vi "EGG Analysis.vi"() -> ()   [LabVIEW 2020]
uses:
  <vilib>/sound2/lvsound2.llb/Sound File Read Open.vi
  <vilib>/sound2/lvsound2.llb/Sound File Read (DBL).vi
  <vilib>/Waveform/WDTOps.llb/WDT Get Waveform Subset DBL.vi
  <vilib>/measure/matone.llb/Extract Multiple Tone Information 1 Chan.vi
  <vilib>/measure/NI_MAPro.lvlib
  <vilib>/Analysis/NI_AALPro.lvlib
panel:
  in  "OK Button":bool
  out "Sample Subset":waveform(dbl)(graph)
  out "Full Sample":waveform(dbl)(graph)
  in  "Cutoff":dbl=0.01 min=0.01 max=0.99 step=0.01
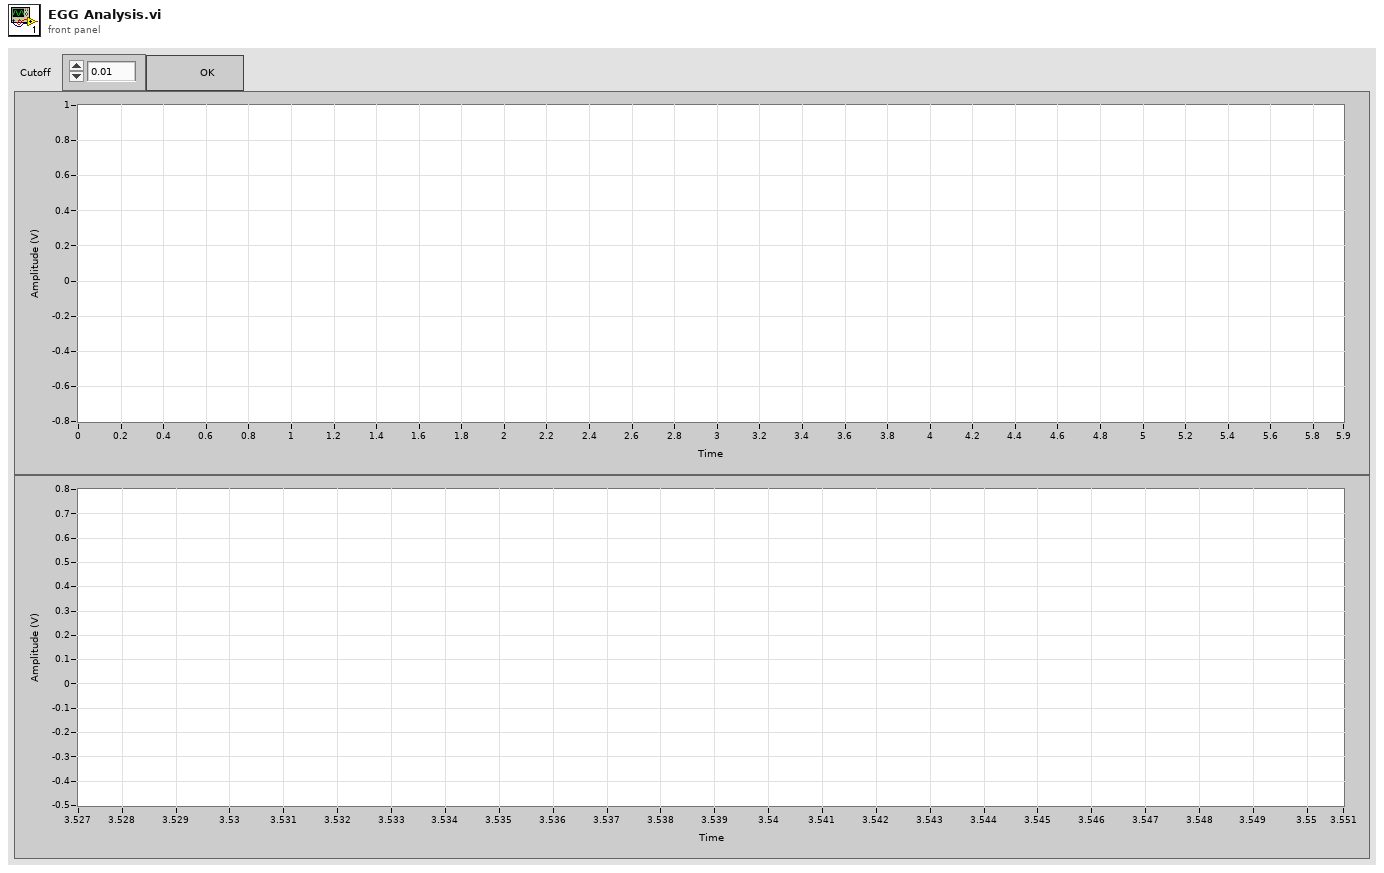
[diagram p1: front panel]
types:
  T1 = typedef "Sound File Refnum.ctl" = refnum<file>
  T2 = cluster{"Name":string, "Color":u32, "Style":u8, "Point Style":u8, "Name Visible":bool, "Allow Drag":bool, "Cursor Mode":u32, "Plot":i32, "Index":i32, "Position":cluster{"X":dbl, "Y":dbl}, "X Scale":u32, "Y Scale":u32, "Watch Plots":i32[], "Watch All Plots":bool, "Plot Area":i32, "Label Offset":cluster{"X":dbl, "Y":dbl}}[]
  T3 = typedef "LVCursorListTypeDef.ctl" = cluster{"Name":string, "Color":u32, "Style":u8, "Point Style":u8, "Name Visible":bool, "Allow Drag":bool, "Cursor Mode":u32, "Plot":i32, "Index":i32, "Position":cluster{"X":dbl, "Y":dbl}, "X Scale":u32, "Y Scale":u32, "Watch Plots":i32[], "Watch All Plots":bool, "Plot Area":i32, "Label Offset":cluster{"X":dbl, "Y":dbl}}[]
  T4 = cluster{"CrsrList[0]":cluster{"Name":string, "Color":u32, "Style":u8, "Point Style":u8, "Name Visible":bool, "Allow Drag":bool, "Cursor Mode":u32, "Plot":i32, "Index":i32, "Position":cluster{"X":dbl, "Y":dbl}, "X Scale":u32, "Y Scale":u32, "Watch Plots":i32[], "Watch All Plots":bool, "Plot Area":i32, "Label Offset":cluster{"X":dbl, "Y":dbl}}, "CrsrList[1]":cluster{"Name":string, "Color":u32, "Style":u8, "Point Style":u8, "Name Visible":bool, "Allow Drag":bool, "Cursor Mode":u32, "Plot":i32, "Index":i32, "Position":cluster{"X":dbl, "Y":dbl}, "X Scale":u32, "Y Scale":u32, "Watch Plots":i32[], "Watch All Plots":bool, "Plot Area":i32, "Label Offset":cluster{"X":dbl, "Y":dbl}}, "CrsrList[2]":cluster{"Name":string, "Color":u32, "Style":u8, "Point Style":u8, "Name Visible":bool, "Allow Drag":bool, "Cursor Mode":u32, "Plot":i32, "Index":i32, "Position":cluster{"X":dbl, "Y":dbl}, "X Scale":u32, "Y Scale":u32, "Watch Plots":i32[], "Watch All Plots":bool, "Plot Area":i32, "Label Offset":cluster{"X":dbl, "Y":dbl}}, "CrsrList[3]":cluster{"Name":string, "Color":u32, "Style":u8, "Point Style":u8, "Name Visible":bool, "Allow Drag":bool, "Cursor Mode":u32, "Plot":i32, "Index":i32, "Position":cluster{"X":dbl, "Y":dbl}, "X Scale":u32, "Y Scale":u32, "Watch Plots":i32[], "Watch All Plots":bool, "Plot Area":i32, "Label Offset":cluster{"X":dbl, "Y":dbl}}, "CrsrList[4]":cluster{"Name":string, "Color":u32, "Style":u8, "Point Style":u8, "Name Visible":bool, "Allow Drag":bool, "Cursor Mode":u32, "Plot":i32, "Index":i32, "Position":cluster{"X":dbl, "Y":dbl}, "X Scale":u32, "Y Scale":u32, "Watch Plots":i32[], "Watch All Plots":bool, "Plot Area":i32, "Label Offset":cluster{"X":dbl, "Y":dbl}}, "CrsrList[5]":cluster{"Name":string, "Color":u32, "Style":u8, "Point Style":u8, "Name Visible":bool, "Allow Drag":bool, "Cursor Mode":u32, "Plot":i32, "Index":i32, "Position":cluster{"X":dbl, "Y":dbl}, "X Scale":u32, "Y Scale":u32, "Watch Plots":i32[], "Watch All Plots":bool, "Plot Area":i32, "Label Offset":cluster{"X":dbl, "Y":dbl}}, "CrsrList[6]":cluster{"Name":string, "Color":u32, "Style":u8, "Point Style":u8, "Name Visible":bool, "Allow Drag":bool, "Cursor Mode":u32, "Plot":i32, "Index":i32, "Position":cluster{"X":dbl, "Y":dbl}, "X Scale":u32, "Y Scale":u32, "Watch Plots":i32[], "Watch All Plots":bool, "Plot Area":i32, "Label Offset":cluster{"X":dbl, "Y":dbl}}, "CrsrList[7]":cluster{"Name":string, "Color":u32, "Style":u8, "Point Style":u8, "Name Visible":bool, "Allow Drag":bool, "Cursor Mode":u32, "Plot":i32, "Index":i32, "Position":cluster{"X":dbl, "Y":dbl}, "X Scale":u32, "Y Scale":u32, "Watch Plots":i32[], "Watch All Plots":bool, "Plot Area":i32, "Label Offset":cluster{"X":dbl, "Y":dbl}}, "CrsrList[8]":cluster{"Name":string, "Color":u32, "Style":u8, "Point Style":u8, "Name Visible":bool, "Allow Drag":bool, "Cursor Mode":u32, "Plot":i32, "Index":i32, "Position":cluster{"X":dbl, "Y":dbl}, "X Scale":u32, "Y Scale":u32, "Watch Plots":i32[], "Watch All Plots":bool, "Plot Area":i32, "Label Offset":cluster{"X":dbl, "Y":dbl}}}
  T5 = cluster{"detected frequency":dbl, "detected amplitude":dbl, "detected phase (deg)":dbl}[]
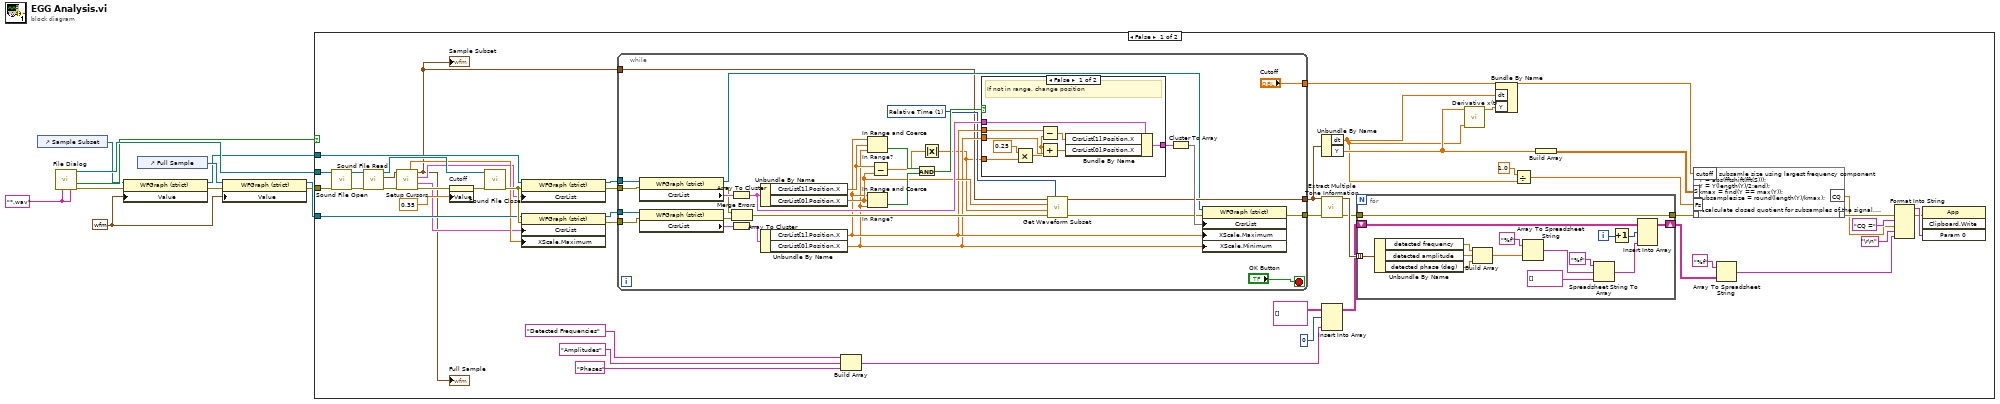
[diagram p0: block diagram]
diagram:
  w1 = waveform(dbl) {"t0"=timestamp(0 s since 1904-01-01), "dt"=1.0, "Y"=[]} ("Waveform")
  w10 = "*.wav" ("pattern (all files)")
  n1 = control-ref of="Sample Subset"() -> (w8:refnum<vi>)
  n2 = call "File Dialog"("pattern (all files)"=w10, "pattern label"=w10) -> ("selected path"=w11:path, "cancelled"=w9:bool, "error out"=w2:errorcluster)  [unwired: 10 in, 1 out]
  n3 = property class="WFGraph (strict)"(reference=w8, error in=w2, "Value"=w1) -> (reference out=w3:refnum<vi>, error out=w4:errorcluster)
  n4 = control-ref of="Full Sample"() -> (w7:refnum<vi>)
  n5 = property class="WFGraph (strict)"(reference=w7, error in=w4, "Value"=w1) -> (reference out=w6:refnum<vi>, error out=w5:errorcluster)
  n6 = case shown="False" w9 {
    tunnel: w11 -> [w58 _]
    tunnel: w5 -> [w57 _]
    tunnel: w3 -> [w42 _]
    tunnel: w6 -> [w41 _]
    frame False {
      n7 = call-poly <vilib>:"Sound File Open.vi"("error in (no error)"=w57, "path"=w58) -> ("error out"=w60:errorcluster, "sound file refnum"=w59:T1)  [unwired: 8 in]
      n8 = call-poly <vilib>:"Sound File Read.vi"("error in (no error)"=w60, "sound file refnum"=w59) -> ("error out"=w46:errorcluster, "data"=w54:waveform(dbl)[], "sound file refnum out"=w53:T1)  [unwired: 5 in, 2 out]
      n9 = call "Setup Cursors.vi"("error in (no error)"=w46, "data"=w54) -> ("error out"=w44:errorcluster, "Cursor List 2"=w33:T2, "Cursor List"=w34:T2, "waveform out"=w32:waveform(dbl), "duration"=w35:dbl)  [unwired: 5 in]
      "Full Sample" <- w32
      "Sample Subset" <- w32
      n10 = property on="Cutoff" class="DigNum (strict)"(error in=w44, "Value"=0.35 ("Cutoff")) -> (error out=w43:errorcluster)  [unwired: 1 in, 1 out]
      n11 = call <vilib>:"Sound File Close.vi"("error in (no error)"=w43, "sound file refnum"=w53) -> ("error out"=w51:errorcluster)  [unwired: 9 in]
      n12 = property on="Property Node" class="WFGraph (strict)"(reference=w42, error in=w51, "CrsrList"=w34) -> (reference out=w49:refnum<vi>, error out=w50:errorcluster)
      n13 = property on="Property Node" class="WFGraph (strict)"(reference=w41, error in=w51, "CrsrList"=w33, "XScale.Maximum"=w35) -> (reference out=w48:refnum<vi>, error out=w47:errorcluster)
      n14 = while {
        tunnel: w32 -> [w77]
        tunnel: [w90] -> w40
        tunnel: ["Cutoff"] -> w52
        tunnel: [w83] -> w39
        tunnel: w50 -> [w82]
        tunnel: w49 -> [w81]
        tunnel: w48 -> [w80]
        tunnel: w47 -> [w79]
        stop <- "OK Button" stop-if-true
        w85 = u16 1 items=["Samples", "Relative Time"] ("start/duration format")
        n15 = property on="Property Node" class="WFGraph (strict)"(reference=w81, error in=w82) -> (reference out=w88:refnum<vi>, error out=w93:errorcluster, "CrsrList"=w105:T3)
        n16 = property on="Property Node" class="WFGraph (strict)"(reference=w80, error in=w79) -> (error out=w92:errorcluster, "CrsrList"=w104:T3)  [unwired: 1 out]
        n17 = Array To Cluster(array=w105) -> (cluster=w100:T4)
        n18 = Array To Cluster(array=w104) -> (cluster=w103:T4)
        n19 = Merge Errors(w93, w92) -> (w91:errorcluster)
        n20 = Unbundle By Name(w100) -> ("CrsrList[1].Position.X"=w95:dbl, "CrsrList[0].Position.X"=w94:dbl)
        n21 = Unbundle By Name(w103) -> ("CrsrList[1].Position.X"=w87:dbl, "CrsrList[0].Position.X"=w86:dbl)
        n22 = In Range and Coerce "In Range?"(upper limit=w87, x=w95, lower limit=w86) -> (In Range?=w99:bool)  [unwired: 1 out]
        n23 = In Range and Coerce "In Range?"(upper limit=w87, x=w94, lower limit=w86) -> (In Range?=w98:bool)  [unwired: 1 out]
        n24 = Subtract(x=w95, y=w94) -> (x-y=w96:dbl)
        n25 = And(x=w99, y=w98) -> (x .and. y?=w97:bool)
        n26 = Absolute Value(x=w96) -> (abs(x)=w76:dbl)
        n27 = case shown="False" w97 {
          tunnel: [w114 w115] -> w101
          tunnel: w100 -> [w113 w115]
          tunnel: w86 -> [w112 _]
          tunnel: w87 -> [w111 _]
          tunnel: w76 -> [w106 _]
          frame False {
            # "If not in range, change position"
            n28 = Multiply(x=0.25, y=w106) -> (x*y=w108:dbl)
            n29 = Subtract(x=w111, y=w108) -> (x-y=w110:dbl)
            n30 = Add(x=w108, y=w112) -> (x+y=w109:dbl)
            n31 = Bundle By Name(cluster=w113, "CrsrList[1].Position.X"=w110, "CrsrList[0].Position.X"=w109) -> (w114:T4)
          }
          frame True {
            # "Cursors are within bounds"
          }
        }
        n32 = call-poly <vilib>:"Get Waveform Subset.vi"("start/duration format"=w85, "error in (no error)"=w91, "duration"=w76, "start samples/time"=w94, "waveform in"=w77) -> ("error out"=w84:errorcluster, "waveform out"=w90:waveform(dbl))  [unwired: 1 in, 2 out]
        n33 = Cluster To Array(cluster=w101) -> (array=w102:T2)
        n34 = property on="Property Node" class="WFGraph (strict)"(reference=w88, error in=w84, "CrsrList"=w102, "XScale.Maximum"=w87, "XScale.Minimum"=w86) -> (error out=w83:errorcluster)  [unwired: 1 out]
      }
      n35 = Build Array("Detected Frequencies", "Amplitudes", "Phases") -> (w20:string[])
      n36 = Unbundle By Name(w40) -> ("dt"=w12:dbl, "Y"=w14:dbl[])
      n37 = call-poly <vilib>:"Extract Multiple Tone Information.vi"("time signal in"=w40, "error in (no error)"=w39) -> ("multiple tone information"=w37:T5, "error out"=w36:errorcluster)  [unwired: 11 in, 1 out]
      n38 = Insert Into Array(array=string[][] [], index (row)=0 ("disabled index (col)"), new element=w20) -> (w19:string[][])  [unwired: 1 in]
      n39 = for {
        tunnel: w37 -> [w75] mode=indexing
        tunnel: w36 -> [w74]
        tunnel: [w74] -> w30
        shift-right: [w72] -> w18
        shift-left: w19 -> [w73]
        i -> [w71]
        n40 = Unbundle By Name(w75) -> ("detected frequency"=w69:dbl, "detected amplitude"=w68:dbl, "detected phase (deg)"=w67:dbl)
        n41 = Build Array(w69, w68, w67) -> (w64:dbl[])
        n42 = Array To Spreadsheet String(array=w64, 3:"%f" ("format string")) -> (spreadsheet string=w65:string)  [unwired: 1 in]
        n43 = Spreadsheet String To Array(format string="%f", spreadsheet string=w65, array type (2D Dbl)=string[] []) -> (array=w62:string[])  [unwired: 1 in]
        n44 = Increment(x=w71) -> (x+1=w61:i32)
        n45 = Insert Into Array(array=w73, index (row)=w61, new element=w62) -> (w72:string[][])  [unwired: 1 in]
      }
      n46 = call <vilib>:"Derivative x(t).vi"("dt"=w12, "X"=w14) -> ("dX/dt"=w13:dbl[])  [unwired: 8 in, 1 out]
      n47 = Bundle By Name("dt"=w12, "Y"=w13) -> ()  [unwired: 1 in, 1 out]
      n48 = Divide(x=1.0, y=w12) -> (x/y=w38:dbl)
      n49 = Build Array(w14) -> (w55:dbl[][])
      n50 = script code="%find subsamle size using largest frequency component\nY = abs(fftshift(fft(S)));\nY = Y(length(Y)/2:end);\nkmax = find(Y == max(Y));\nsubsamplesize = round(length(Y)/kmax);\n\n%calculate closed quotient for subsamples of the signal, \n%then find the average for the whole signal\nsubsamples = ceil(length(S)/subsamplesize);\ncq = 0; %running total of closed quotient for each subsample\nfor i = 1:subsamples\n    starti = ((i-1)*subsamplesize)+1;\n    endi = i*subsamplesize;\n    if(endi <= length(S))\n        s = S(starti:endi);\n    else\n        s = S(starti:end);\n    end\n    minval = min(s);\n    s = s - minval;\n    maxval = max(s);\n    closed = length(find(s < (maxval*cutoff)));\n    cq = cq + (closed/length(s));\nend\n\n%calculate average closed quotient for whole signal\nCQ = cq/subsamples;"("??"=w30, "S"=w55, "Fs"=w38, "cutoff"=w52) -> ("??"=w31:errorcluster, "CQ"=w28:dbl)
      n51 = Array To Spreadsheet String(array=w18, 3:"%f" ("format string")) -> (spreadsheet string=w22:string)  [unwired: 1 in]
      n52 = Format Into String(error in=w31, "CQ =", w28, "\r\n", w22) -> (resulting string=w16:string, error out=w15:errorcluster)  [unwired: 2 in]
      n53 = invoke class="App" method="Clipboard.Write"(error in=w15, "Param 0"=w16) -> ()  [unwired: 2 in, 4 out]
    }
    frame True {
    }
  }
